vi "Motion-IntializeNoSplash.vi"(8 "error in (no error)":errorcluster, 11 "Motion-ControlAll in":refnum<class "Motion-ControlAll.lvclass">) -> (0 "error out":errorcluster, 3 "Motion-ControlAll out":refnum<class "Motion-ControlAll.lvclass">)   [LabVIEW 2013, in "Motion-ControlAll.lvclass"]
uses:
  Motion-ControlAll.lvclass
  Motion-ControlAll.lvclass/Motion-ControlAll.ctl
  <vilib>/addons/_LabVIEW Style Book/Utilities/Style Book Utilities.lvlib
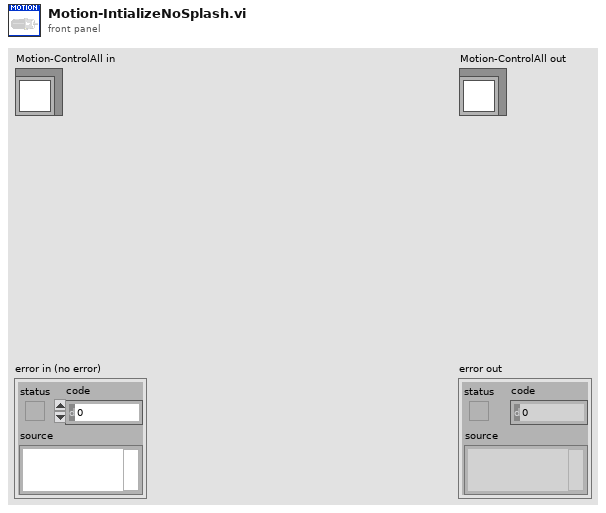
[diagram p1: front panel]
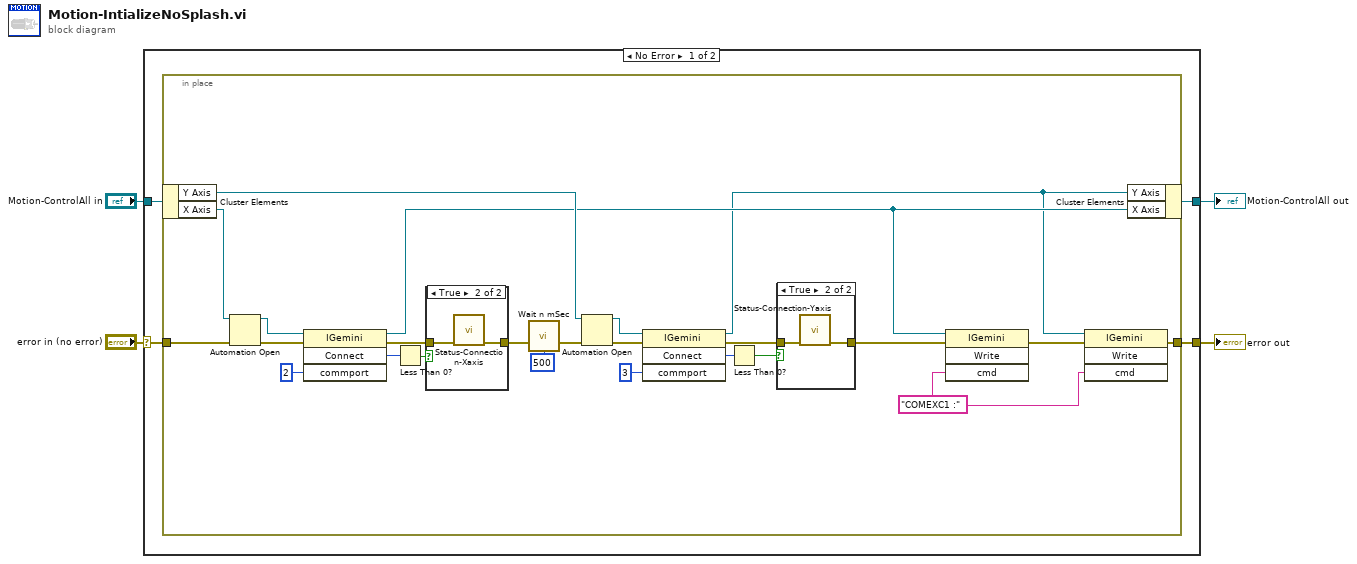
[diagram p0: block diagram]
diagram:
  n1 = case shown="No Error" "error in (no error)" {
    selector: "error in (no error)" -> [w7 w40]
    tunnel: [w6 w40] -> w1
    tunnel: [w5 w39] -> w3
    tunnel: "Motion-ControlAll in" -> [w8 w39]
    frame No Error {
      n2 = in-place {
        in-place-border: w7 -> [w32]
        in-place-border: [w23] -> w6
        w25 = "COMEXC1 :" ("cmd")
        n3 = in-place-cluster #1(w8) -> ("Y Axis"=w14:refnum<k7>, "X Axis"=w24:refnum<k7>)
        n4 = Automation Open(error in (no error)=w32, Automation Refnum=w24) -> (Automation Refnum=w29:refnum<k7>, error out=w30:errorcluster)  [unwired: 2 in]
        n5 = invoke class="IGemini" method="Connect"(reference=w29, error in=w30, "commport"=i16 2) -> (reference out=w13:refnum<k7>, error out=w28:errorcluster, "Connect"=w27:i16)  [unwired: 1 in, 1 out]
        n6 = Less Than 0?(x=w27) -> (x < 0?=w22:bool)
        n7 = case shown="True" w22 {
          tunnel: w28 -> [w36 w38]
          tunnel: [w36 w37] -> w11
          frame False {
          }
          frame True {
            n8 = call "Status-Connection-Xaxis.vi"("error in"=w38) -> ("error out"=w37:errorcluster)  [unwired: 10 in]
          }
        }
        n9 = call <vilib>:"Wait n mSec.vi"("error in (no error)"=w11, "Milliseconds to Wait (500)"=u32 500) -> ("error out"=w10:errorcluster)  [unwired: 13 in]
        n10 = Automation Open(error in (no error)=w10, Automation Refnum=w14) -> (Automation Refnum=w18:refnum<k7>, error out=w19:errorcluster)  [unwired: 2 in]
        n11 = invoke class="IGemini" method="Connect"(reference=w18, error in=w19, "commport"=i16 3) -> (reference out=w12:refnum<k7>, error out=w16:errorcluster, "Connect"=w21:i16)  [unwired: 1 in, 1 out]
        n12 = Less Than 0?(x=w21) -> (x < 0?=w17:bool)
        n13 = case shown="True" w17 {
          tunnel: w16 -> [w33 w35]
          tunnel: [w33 w34] -> w15
          frame False {
          }
          frame True {
            n14 = call "Status-Connection-Yaxis.vi"("error in"=w35) -> ("error out"=w34:errorcluster)  [unwired: 10 in]
          }
        }
        n15 = invoke class="IGemini" method="Write"(reference=w13, error in=w15, "cmd"=w25) -> (error out=w26:errorcluster)  [unwired: 1 in, 3 out]
        n16 = invoke class="IGemini" method="Write"(reference=w12, error in=w26, "cmd"=w25) -> (error out=w23:errorcluster)  [unwired: 1 in, 3 out]
        n17 = in-place-cluster #1("Y Axis"=w12, "X Axis"=w13) -> (w5:refnum<class "Motion-ControlAll.lvclass">)
      }
    }
    frame Error {
    }
  }
  "error out" <- w1
  "Motion-ControlAll out" <- w3
